vi "INFO.vi"(6 "Message":string, 8 "error in":errorcluster) -> (0 "error out":errorcluster)   [LabVIEW 2024, in "hse-logger.lvlib"]
doc: "Logs a message and the content of the error-cluster.\nAn error on the \"error in\" terminal is duplicated to the \"error dup\" terminal.\n\nDoes not return logging errors!\n\n____\nHAMPEL SOFTWARE ENGINEERING v2.2.2 (2025-01-16 15:41)"
uses:
  <vilib>/Hampel Software Engineering/HSE Logger/hse-logger.lvlib
  <vilib>/Utility/error.llb/Error Cluster From Error Code.vi
  <vilib>/Hampel Software Engineering/HSE Logger/Logger/Logger.lvclass
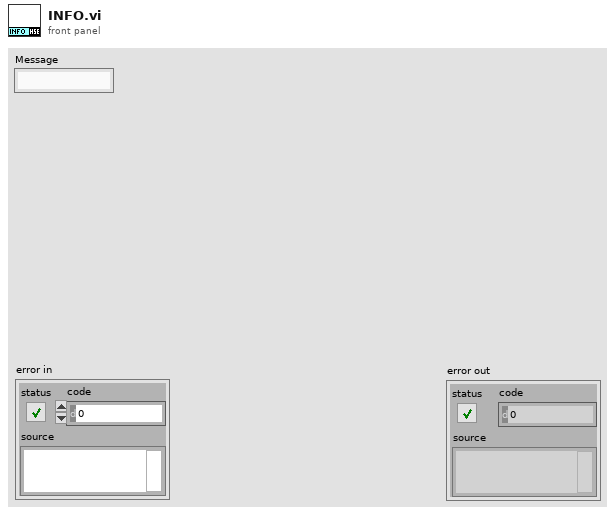
[diagram p1: front panel]
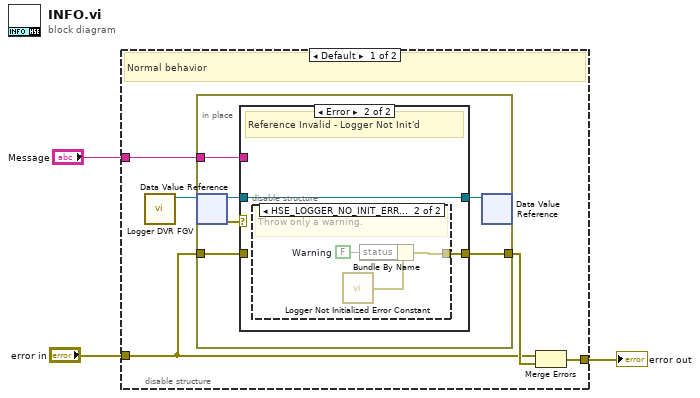
[diagram p0: block diagram]
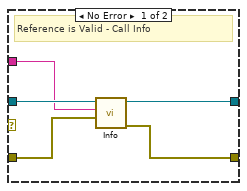
[diagram p2: hidden frame]
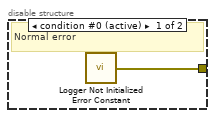
[diagram p3: hidden frame]
diagram:
  n1 = disable-structure shown="Default" {
    disable-tunnel: [w8 w26] -> w3
    disable-tunnel: "Message" -> [w7 _]
    disable-tunnel: "error in" -> [w4 w26]
    frame condition #0 (active) {
      # "Normal behavior"
      n2 = call <vilib>:"Logger DVR FGV.vi"() -> ("Logger DVR"=w6:refnum<data-value>)  [unwired: 10 in, 1 out]
      n3 = in-place {
        in-place-border: w7 -> [w13]
        in-place-border: [w12] -> w5
        in-place-border: w4 -> [w9]
        n4 = in-place-dvr #1(w6) -> (w14:refnum<class "Logger.lvclass">, w10:errorcluster)
        n5 = case shown="Error" w10 {
          tunnel: w14 -> [w19 w21]
          tunnel: w13 -> [w18 _]
          tunnel: [w17 w20] -> w12
          tunnel: [w16 w21] -> w11
          tunnel: w9 -> [w15 _]
          frame No Error {
            # "Reference is Valid - Call Info"
            n6 = call-dynamic "Info.vi"("Error to Log"=w15, "Message"=w18, "Logger in"=w19) -> ("error out"=w17:errorcluster, "Logger out"=w16:refnum<class "Logger.lvclass">)  [unwired: 7 in]
          }
          frame Error {
            # "Reference Invalid - Logger Not Init'd"
            n7 = disable-structure shown="HSE_LOGGER_NO_INIT_ERROR==True" {
              disable-tunnel: [w22 w24] -> w20
              frame condition #0 (active) {
                # "Normal error"
                n8 = call <vilib>:"Logger Not Initialized Error Constant.vi"() -> ("Logger Not Initialized Error"=w22:errorcluster)
              }
              frame condition #1 {
                w23 = FALSE  # Warning
                # "Throw only a warning."
                n9 = call <vilib>:"Logger Not Initialized Error Constant.vi"() -> ("Logger Not Initialized Error"=w25:errorcluster)
                n10 = Bundle By Name(cluster=w25, "status"=w23) -> (w24:errorcluster)
              }
            }
          }
        }
        n11 = in-place-dvr #1(w11) -> ()  [unwired: 2 out]
      }
      n12 = Merge Errors(w4, w5) -> (w8:errorcluster)
    }
    frame condition #1 {
      # "Logging disabled"
    }
  }
  "error out" <- w3
